vi "Counter (Buffered) - Continuous Output.vi"() -> ()   [LabVIEW 2022 SP3]
doc: "This example demonstrates how to continuously generate digital pulses using a counter output."
uses:
  <vilib>/Utility/error.llb/DialogType.ctl
  <vilib>/DAQmx/write.llb/DAQmx Write (Counter 1D Time 1Chan NSamp).vi
  <vilib>/DAQmx/create/channels.llb/DAQmx Create Channel (CO-Pulse Generation-Frequency).vi
  <vilib>/DAQmx/configure/timing.llb/DAQmx Timing (Implicit).vi
  <vilib>/DAQmx/configure/timing.llb/DAQmx Timing (Sample Clock).vi
  <vilib>/DAQmx/miscellaneous.llb/DAQmx Fill In Error Info.vi
  <resource>/objmgr/daqmx.rc
panel:
  in  "Output Array":cluster{"High Time":dbl, "Low Time":dbl}[](array[cluster])=[{"High Time"=1.0, "Low Time"=1.0}, {"High Time"=0.5, "Low Time"=0.5}]
  in  "Timing Type":enum32{"Implicit", "External Clock"}(tab)
  in  "Sample Clock Source":tag="/Dev1/PFI0"
  in  "Sample Rate":dbl=1000.0
  in  "Output Terminal":tag="/Dev1/PFI12"
  in  "Stop":bool
  in  "Counter":tag="Dev1/ctr0"
  # "Channel Settings"
  # "Output Buffer"
  # "Timing Settings"
  # "With implicit timing, each pulse will be generated exactly once before the counter output moves on to the next sample in the buffer."
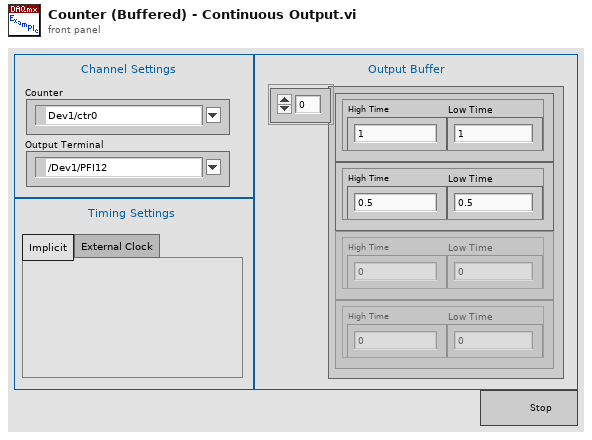
[diagram p1: front panel]
types:
  T1 = typedef "DialogType.ctl" = u16
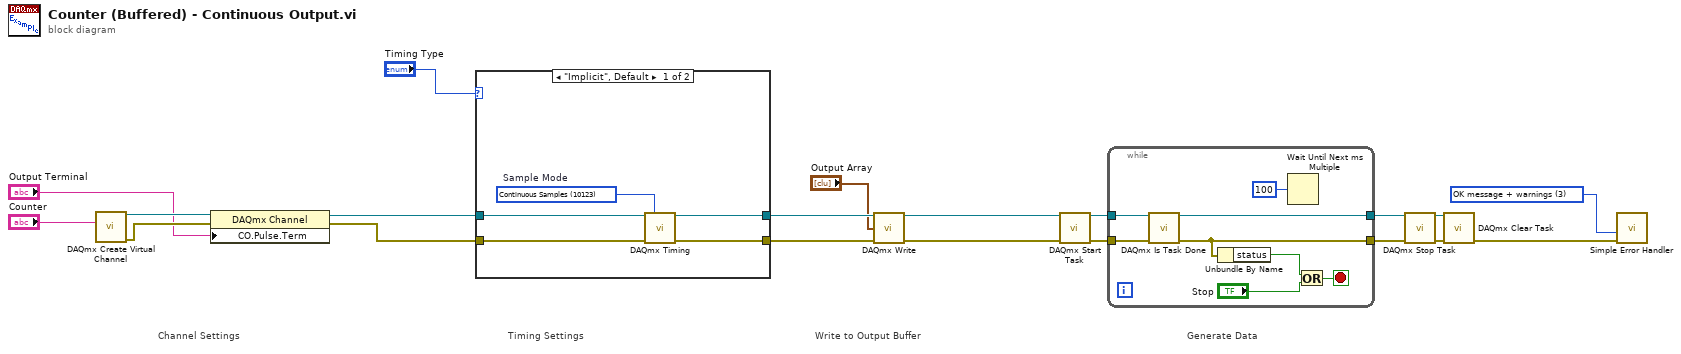
[diagram p0: block diagram]
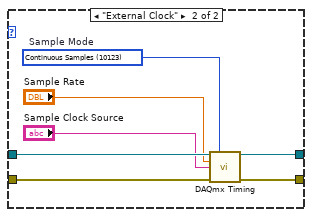
[diagram p2: hidden frame]
diagram:
  w1 = T1 3 items=["no dialog", "OK message", "continue or stop message", "OK message + warnings", "continue/stop + warnings"] ("type of dialog (OK msg:1)")
  # "Generate Data"
  # "Write to Output Buffer"
  # "Timing Settings"
  # "Channel Settings"
  n1 = call-poly <vilib>:"DAQmx Create Virtual Channel.vi"("counter"="Counter") -> ("task out"=w16:refnum<k21>, "error out"=w15:errorcluster)  [unwired: 13 in]
  n2 = property class="DAQmx Channel"(reference=w16, error in=w15, "CO.Pulse.Term"="Output Terminal") -> (reference out=w12:refnum<k21>, error out=w13:errorcluster)
  n3 = case shown="\"Implicit\", Default" "Timing Type" {
    tunnel: w13 -> [w24 w30]
    tunnel: w12 -> [w23 w29]
    tunnel: [w22 w31] -> w11
    tunnel: [w21 w32] -> w10
    frame "Implicit", Default {
      w25 = 10123 items=["Finite Samples"=10178, "Continuous Samples"=10123, "Hardware Timed Single Point"=12522]  # Sample Mode
      n4 = call-poly <vilib>:"DAQmx Timing.vi"("task/channels in"=w23, "sample mode"=w25, "error in"=w24) -> ("task out"=w21:refnum<k21>, "error out"=w22:errorcluster)  [unwired: 11 in]
    }
    frame "External Clock" {
      w26 = 10123 items=["Finite Samples"=10178, "Continuous Samples"=10123, "Hardware Timed Single Point"=12522]  # Sample Mode
      n5 = call-poly <vilib>:"DAQmx Timing.vi"("task/channels in"=w29, "sample mode"=w26, "rate"="Sample Rate", "source"="Sample Clock Source", "error in"=w30) -> ("task out"=w32:refnum<k21>, "error out"=w31:errorcluster)  [unwired: 9 in]
    }
  }
  n6 = call-poly <vilib>:"DAQmx Write.vi"("task/channels in"=w10, "data"="Output Array", "error in"=w11) -> ("task out"=w9:refnum<k21>, "error out"=w8:errorcluster)  [unwired: 10 in, 1 out]
  n7 = call <vilib>:"DAQmx Start Task.vi"("task/channels in"=w9, "error in"=w8) -> ("task out"=w20:refnum<k21>, "error out"=w19:errorcluster)  [unwired: 12 in]
  n8 = while {
    tunnel: w20 -> [w40]
    tunnel: w19 -> [w39]
    tunnel: [w36] -> w2
    tunnel: [w37] -> w3
    stop <- w38 stop-if-true
    n9 = call <vilib>:"DAQmx Is Task Done.vi"("task/channels in"=w40, "error in"=w39) -> ("task out"=w37:refnum<k21>, "error out"=w36:errorcluster)  [unwired: 11 in, 1 out]
    n10 = Unbundle By Name(w36) -> ("status"=w35:bool)
    n11 = Wait Until Next ms Multiple(millisecond multiple=u32 100) -> ()  [unwired: 1 out]
    n12 = Or(x=w35, y="Stop") -> (x .or. y?=w38:bool)
  }
  n13 = call <vilib>:"DAQmx Stop Task.vi"("task/channels in"=w3, "error in"=w2) -> ("task out"=w5:refnum<k21>, "error out"=w4:errorcluster)  [unwired: 12 in]
  n14 = call <vilib>:"DAQmx Clear Task.vi"("task in"=w5, "error in"=w4) -> ("error out"=w18:errorcluster)  [unwired: 13 in]
  n15 = call <vilib>:"Simple Error Handler.vi"("type of dialog (OK msg:1)"=w1, "error in (no error)"=w18) -> ()  [unwired: 3 in, 5 out]
